vi "PID_Discipline_WithoutSystem_X72_Single.vi"(0 "SR620_No.1_Port":refnum<visa-resource-name>="GPIB0::20::INSTR", 1 "Channel (1: A)":i32(ring)=1 items=["Ext Input", "A", "B"], 2 "SR620_No.1 (1: REF)":i32(ring) items=["A", "B", "REF", "A / B"], 3 "Meas. Mode (0: Time)":i32(ring) items=["Time", "Width", "Rise / Fall Time", "Frequency", "Period", "Phase", "Count"], 4 "Arming Mode (0: +/-time)":i32(ring)=1 items=["+/-time", "+time", "1 period", "0.01s gate", "0.1s gate", "1.0s gate", "ext trig +/- time", "ext trig +time", "ext gate/+ time/hldf", "ext triggered 1 period", "ext triggered .01s gate", "ext triggered 0.1s gate", "ext triggered 1.0s gate"], 5 "Gate Time (Auto)":dbl(ring) items=["Auto"=0.0, "1E-6"=1e-06, "2E-6"=2e-06, "5E-6"=5e-06, "1E-5"=1e-05, "2E-5"=2e-05, "5E-5"=5e-05, "1E-4"=0.0001, "2E-4"=0.0002, "5E-4"=0.0005, "1E-3"=0.001, "2E-3"=0.002, "5E-3"=0.005, ".01"=0.01, ".02"=0.02, ".05"=0.05, ".1"=0.1, ".2"=0.2, ".5"=0.5, "1"=1.0, "2"=2.0, "5"=5.0, "10"=10.0, "20"=20.0, "50"=50.0, "100"=100.0, "200"=200.0, "500"=500.0], 6 "Sample Size (1)":u32(ring)=1 items=["1"=1, "2"=2, "5"=5, "10"=10, "20"=20, "50"=50, "100"=100, "200"=200, "500"=500, "1000"=1000, "2000"=2000, "5000"=5000, "10000"=10000, "20000"=20000, "50000"=50000, "100000"=100000, "200000"=200000, "500000"=500000, "1000000"=1000000], 7 "SR620_No.1_error in (no error)1":errorcluster, 8 "Input Termination_ (0: 50 Ohms)":i32(ring) items=["50 Ohms", "1 Mohm", "UHF Prescalers"], 9 "Timeout (25000 ms)":u32=1000 step=1000, 10 "Coupling (F: DC)":bool, 11 "Ref Out (1: TTL)":i32(ring)=1 items=["ECL", "TTL"], 12 "Auto Trigger Level (True)":bool, 14 "Trigger Level (0.00 V)":dbl=1.0, 16 "Trigger Slope (T: Positive)":bool=TRUE) -> (20 "SR620_No.1":refnum<visa-resource-name>="GPIB0::20::INSTR", 27 "SR620_No1 error out":errorcluster)   [LabVIEW 2014]
doc: "Provides an example of how to use the SR620 subVIs programmatically."
uses:
  <vilib>/addons/control/pid/pid.llb/PID (DBL).vi
  <vilib>/Utility/file.llb/Write To Spreadsheet File (DBL).vi
  <vilib>/Instr/_visa.llb/VISA Configure Serial Port (Instr).vi
  <vilib>/addons/control/pid/NI_PID_pid.lvlib
panel:
  out "本地测量钟差":dbl[](graph)=[7593300.0, 241.375901, 241.375903, 241.375876, 241.375868, 241.375803, 241.375857, 241.375887, 241.375852, 241.37583800000002, 241.37586299999998]
  in  "开始绘图":bool
  in  "delimiter (\\n)":string="\n" caption="数据分隔符(\\n)"
  in  "文件路径: single":path=path "C:/Users/Administrator/Desktop/PID_Discipline_WithoutSystem_X72_Single/single_read_data.txt"
  out "是否清零":dbl
  out "钟差改变量":dbl format="%#_10g"
  in  "驯服阈值(ns)":dbl=100.0
  out "驯服":bool
  out "当前粗调调整量（100ns）":i64
  in  "FPGA串口地址":refnum<visa-resource-name>="COM6"
  out "串口读取数值":i64
  out "读取缓冲区 （16进制）":string
  out "写入字符串2":string
  out "写入字符串1":string="0"
  out "最终粗调调整量（100ns）":i64
  in  "output range":cluster{"output high":dbl, "output low":dbl}={"output high"=400.0, "output low"=-400.0} caption="输出范围" {"output low" format="%.2f"; "output high" format="%.2f"}
  in  "PID gains":T1={"proportional gain (Kc)"=0.5, "integral time (Ti, min)"=0.0, "derivative time (Td, min)"=0.0} caption="PID增益" {"derivative time (Td, min)" format="%.3f"; "integral time (Ti, min)" format="%.3f"; "proportional gain (Kc)" format="%.3f"}
  out "反馈值":dbl format="%#.6f"
  in  "setpoint":dbl caption="设定值" format="%.3f"
  out "dt out (s)":dbl=1.0000000474974513 caption="dt输出(s)" format="%.3f"
  out "output":dbl caption="PID输出" format="%#.6f"
  in  "baud rate (9600) 2":u32=57600 caption="波特率(9600)"
  in  "VISA resource name 2":refnum<visa-resource-name>="COM3" caption="VISA资源名称"
  out "错误输出 2":errorcluster caption="错误输出"
  in  "baud rate (9600) 1":u32=57600 caption="波特率(9600)"
  in  "VISA resource name 1":refnum<visa-resource-name>="COM3" caption="VISA资源名称"
  out "错误输出 1":errorcluster caption="错误输出"
  out "串口工作":bool
  out "命令":string
  out "SR620_Delta_T":dbl format="%.12f"
  in  "等待时间（ms)":u32=1000
  out "总计数值":i32
  # "串口"
  # "数据处理"
  # "钟差调整量（ns）"
  # "数据显示及波形显示区域"
  # "公共调节区域"
  # "分别设置区域"
  # "Delta_T"
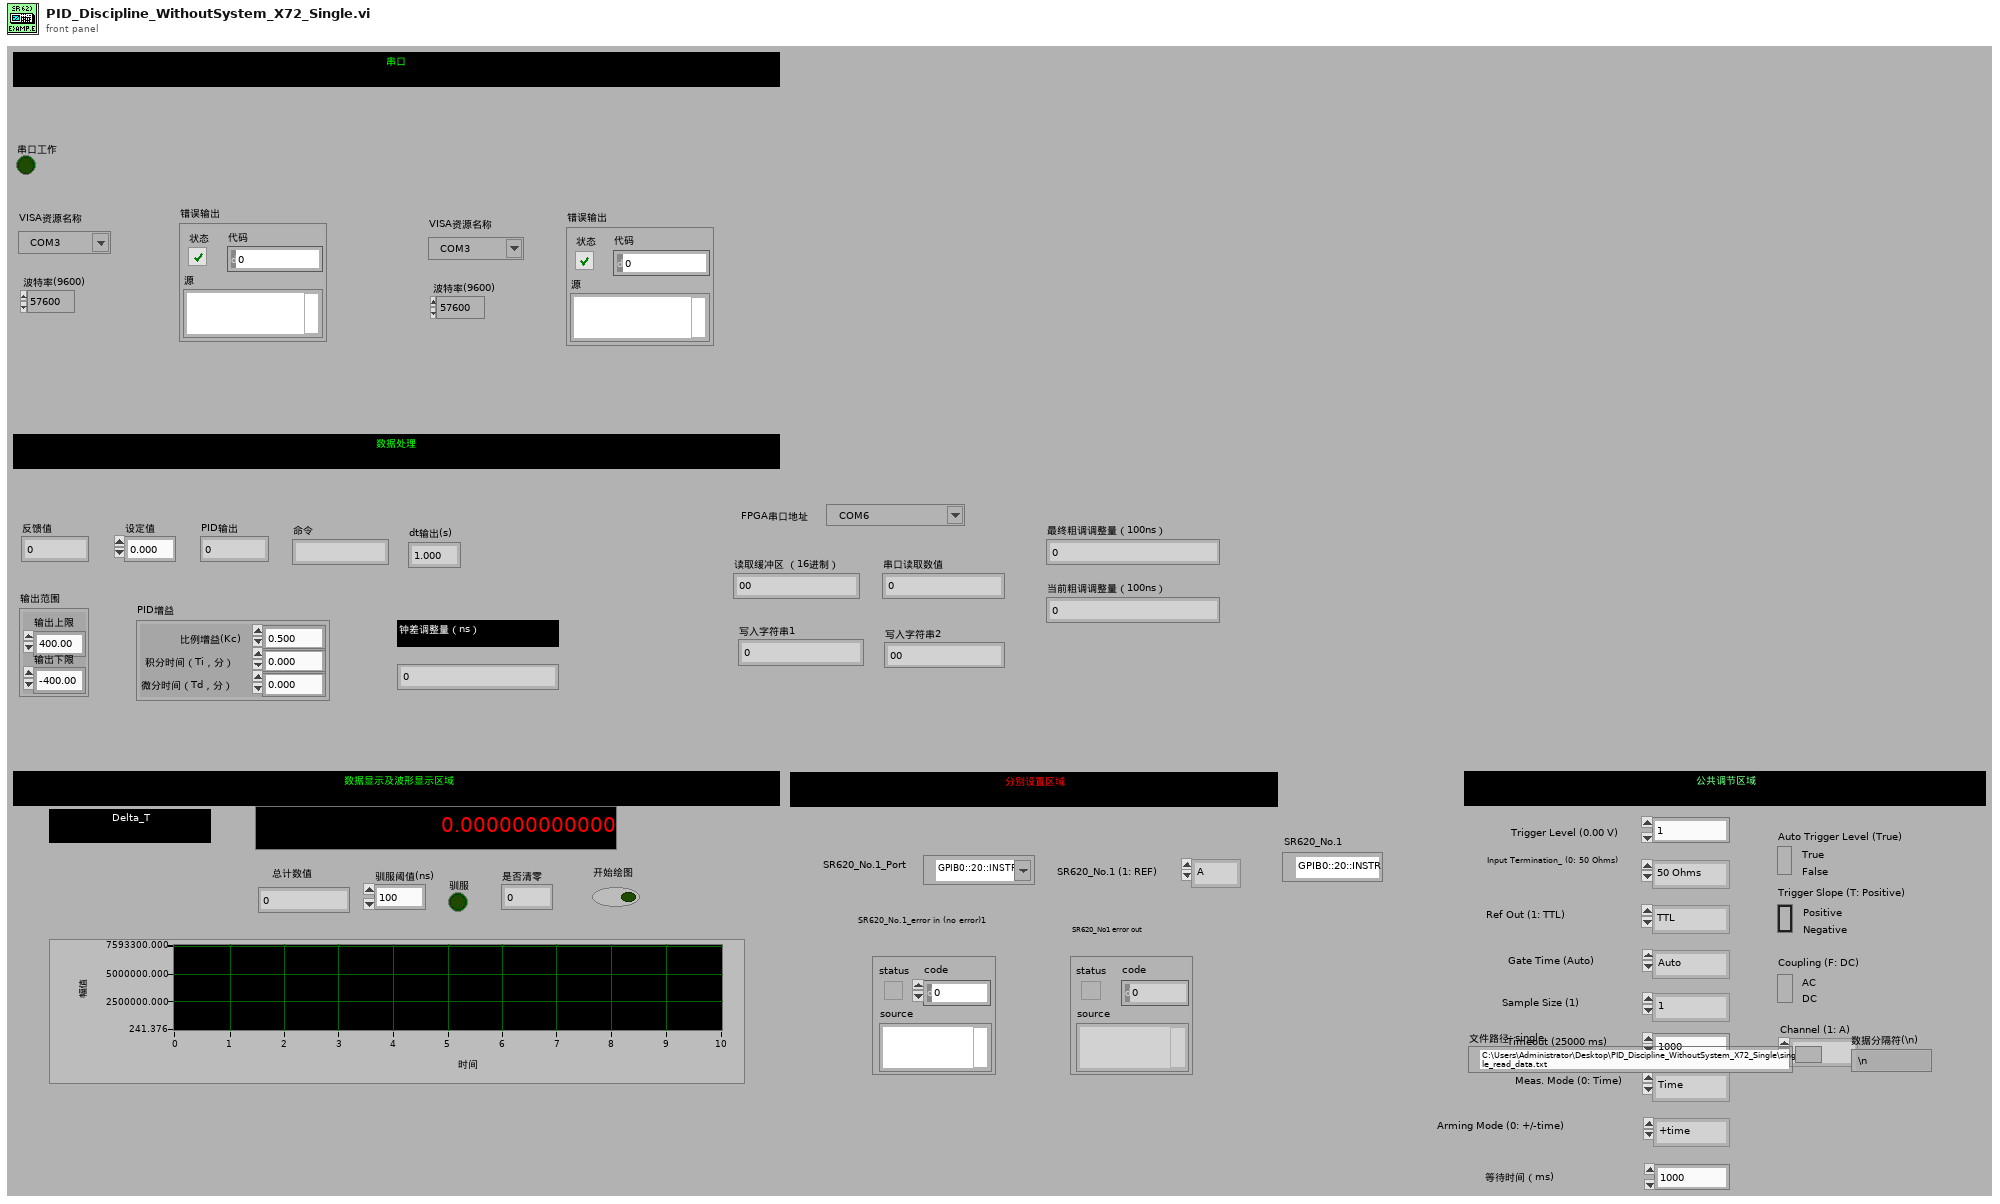
[diagram p1: front panel]
types:
  T1 = cluster{"proportional gain (Kc)":dbl, "integral time (Ti, min)":dbl, "derivative time (Td, min)":dbl}
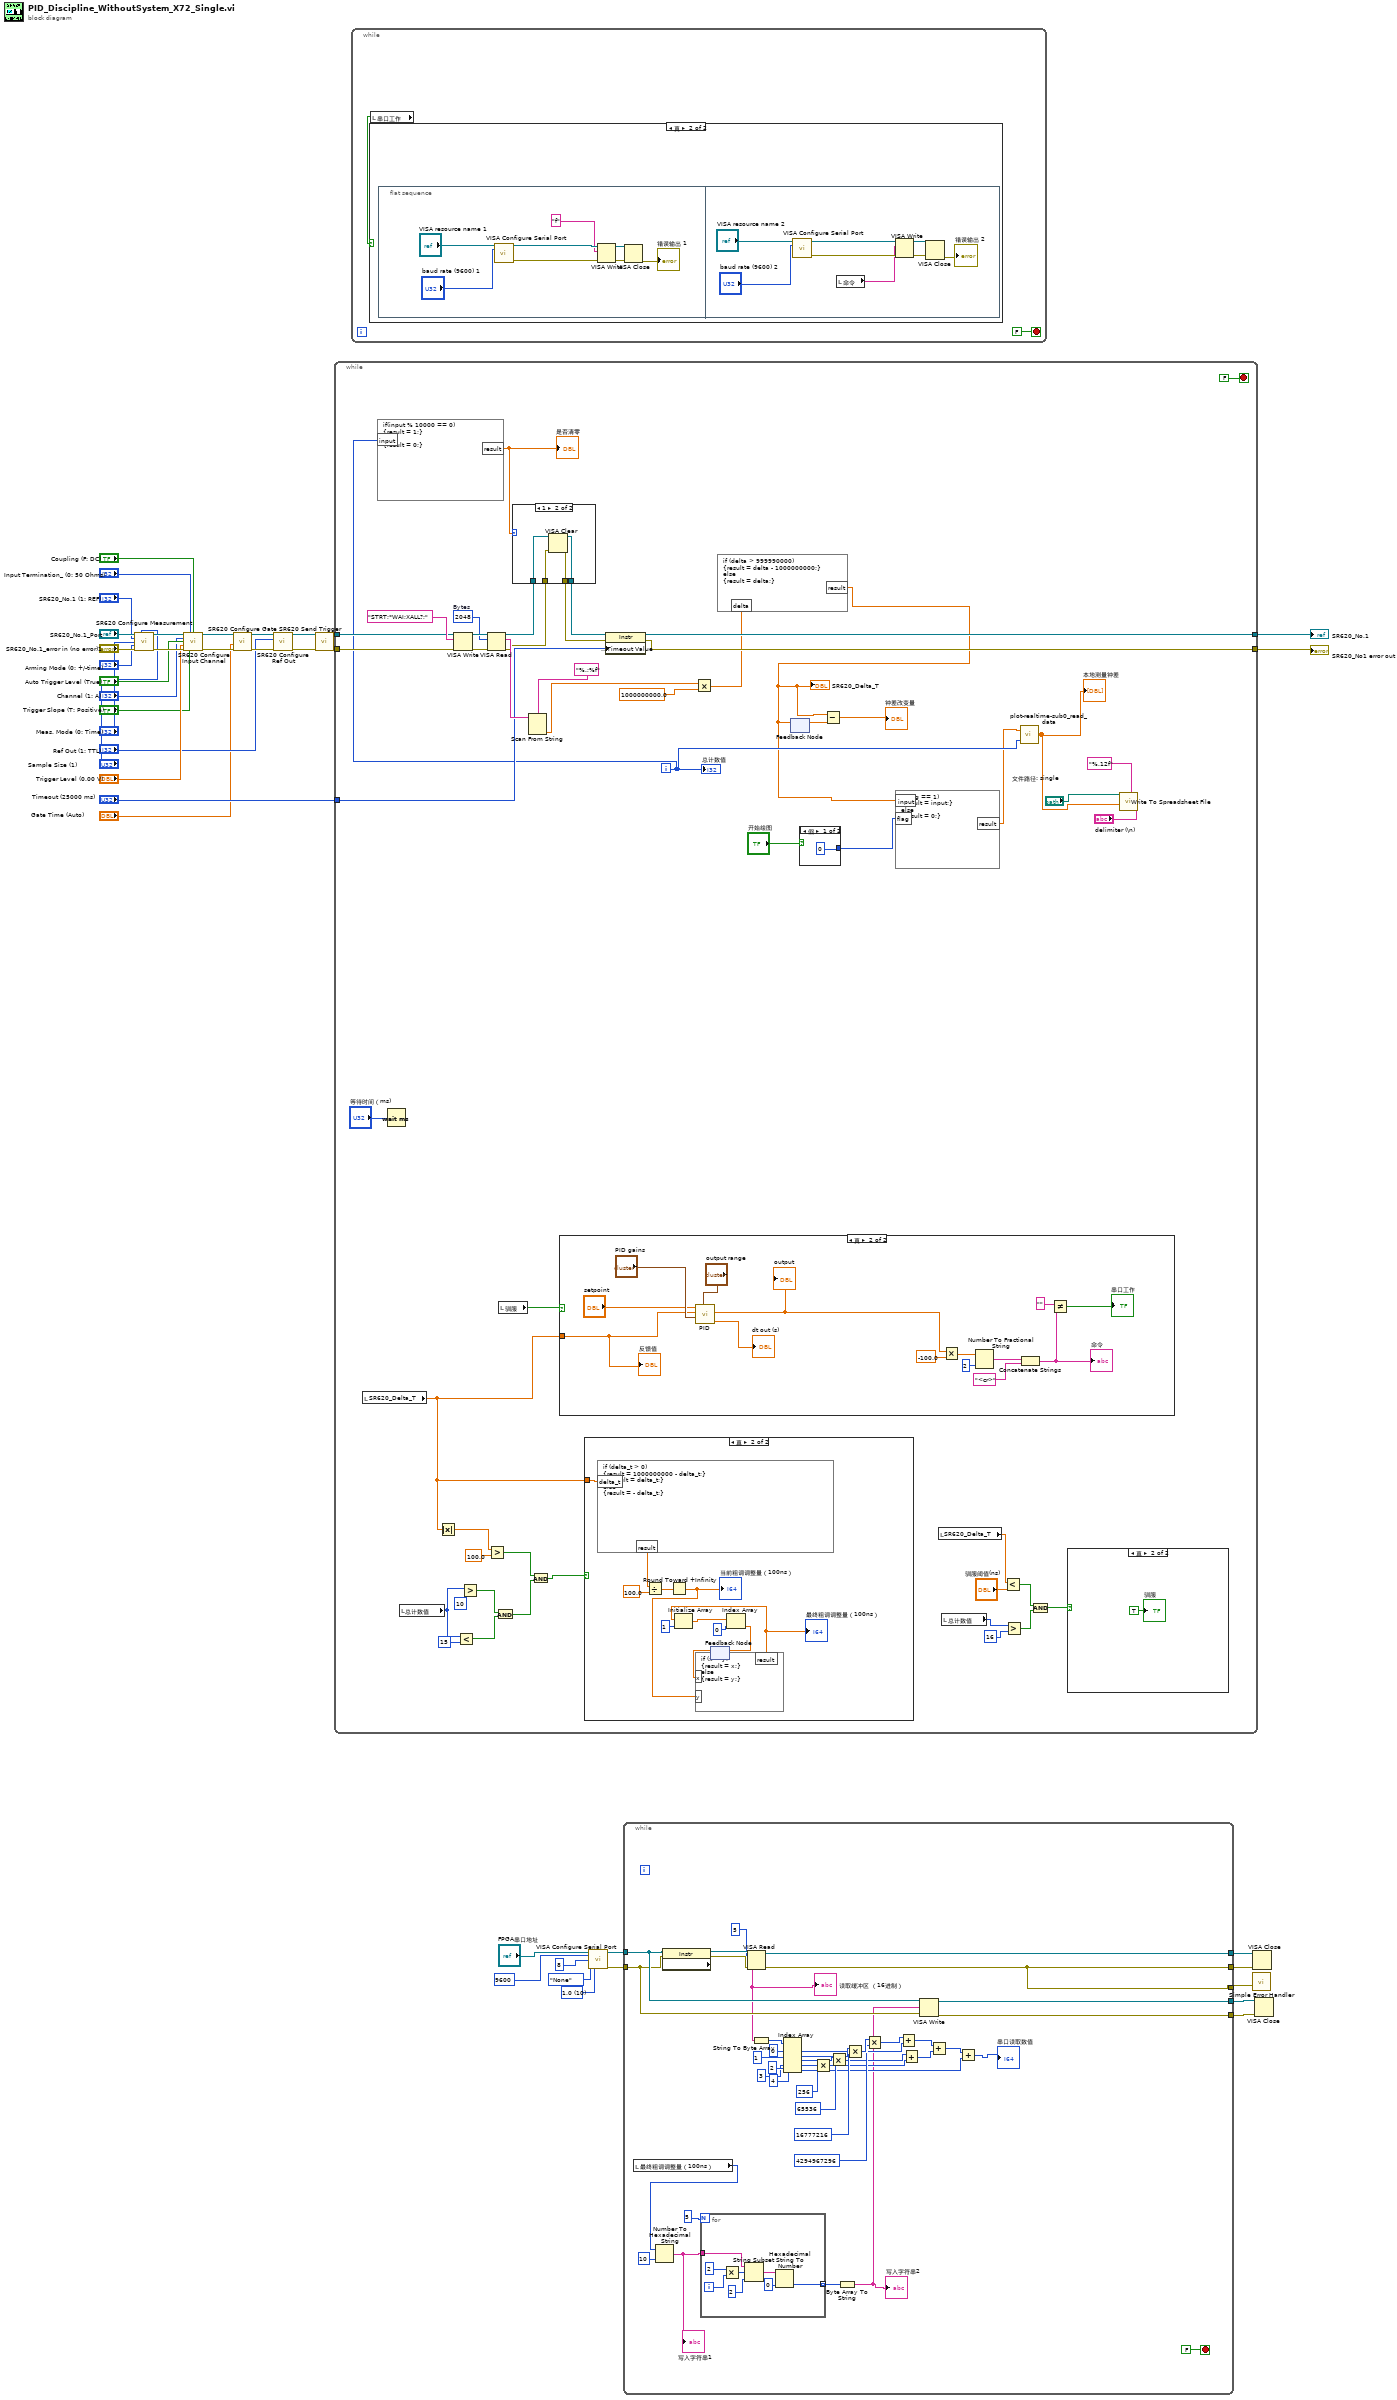
[diagram p0: block diagram]
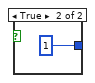
[diagram p3: hidden frame]
diagram:
  w20 = u16 10 items=["1.0"=10, "1.5"=15, "2.0"=20] ("stop bits (10: 1 bit)")
  n1 = call "SR620 Configure Measurement.vi"("VISA session"="SR620_No.1_Port", "Sample Size (1)"="Sample Size (1)", "Source (2: REF)"="SR620_No.1 (1: REF)", "Measurement Mode (0: Time)"="Meas. Mode (0: Time)", "Arming Mode (0: +/-time)"="Arming Mode (0: +/-time)", "error in (no error)"="SR620_No.1_error in (no error)1") -> ("dup VISA session"=w30:refnum<visa-resource-name>, "error out"=w28:errorcluster)  [unwired: 8 in]
  n2 = call "SR620 Configure Input Channel.vi"("VISA session"=w30, "Input Termination (0: 50 Ohms)"="Input Termination_ (0: 50 Ohms)", "Coupling (F: DC)"="Coupling (F: DC)", "Channel (1: A)"="Channel (1: A)", "Auto Trigger Level (True)"="Auto Trigger Level (True)", "Trigger Level (0.00 V)"="Trigger Level (0.00 V)", "error in (no error)"=w28, "Trigger Slope (T: Positive)"="Trigger Slope (T: Positive)") -> ("dup VISA session"=w29:refnum<visa-resource-name>, "error out"=w27:errorcluster)  [unwired: 6 in]
  n3 = call "SR620 Configure Gate.vi"("error in (no error)"=w27, "Gate Time (Auto)"="Gate Time (Auto)", "VISA session"=w29) -> ("error out"=w32:errorcluster, "dup VISA session"=w31:refnum<visa-resource-name>)  [unwired: 5 in]
  n4 = call "SR620 Configure Ref Out.vi"("error in (no error)"=w32, "Amplitude: Ref Output (1: TTL)"="Ref Out (1: TTL)", "VISA session"=w31) -> ("error out"=w33:errorcluster, "dup VISA session"=w34:refnum<visa-resource-name>)  [unwired: 3 in]
  n5 = call "SR620 Send Trigger.vi"("VISA session"=w34, "error in (no error)"=w33) -> ("dup VISA session"=w38:refnum<visa-resource-name>, "error out"=w37:errorcluster)  [unwired: 12 in]
  n6 = while "While循环" {
    tunnel: w38 -> [w84]
    tunnel: w37 -> [w83]
    tunnel: "Timeout (25000 ms)" -> [w60]
    tunnel: [w82] -> w25
    tunnel: [w81] -> w24
    i -> [w48]
    stop <- FALSE stop-if-true
    w88 = u32 2048  # Bytes
    n7 = local read "SR620_Delta_T"() -> (w55:dbl)
    n8 = formula code="if(input % 10000 == 0)\n{result = 1;}\nelse\n{result = 0;}"("input"=w48) -> ("result"=w49:dbl)
    "是否清零" <- w49
    n9 = Wait (ms)(milliseconds to wait="等待时间（ms)") -> ()  [unwired: 1 out]
    n10 = local read "总计数值"() -> (w75:i32)
    n11 = Absolute Value(x=w55) -> (abs(x)=w61:dbl)
    n12 = VISA Write(VISA resource name=w84, write buffer="STRT;*WAI;XALL?;" ("write buffer (\"\")"), error in (no error)=w83) -> (VISA resource name out=w89:refnum<visa-resource-name>, error out=w90:errorcluster)  [unwired: 1 out]
    n13 = Less?(x=w75, y=15) -> (x < y?=w72:bool)
    n14 = Greater?(x=w75, y=10) -> (0:w73:bool)
    n15 = VISA Read(VISA resource name=w89, byte count=w88, error in (no error)=w90) -> (VISA resource name out=w54:refnum<visa-resource-name>, read buffer=w85:string, error out=w52:errorcluster)  [unwired: 1 out]
    n16 = Greater?(x=w61, y=100.0) -> (0:w71:bool)
    n17 = And(x=w73, y=w72) -> (x .and. y?=w70:bool)
    n18 = local read "驯服"() -> (w63:bool)
    n19 = case shown="1" w49 {
      tunnel: w54 -> [w94 w98]
      tunnel: [w94 w97] -> w53
      tunnel: w52 -> [w93 w96]
      tunnel: [w93 w95] -> w51
      frame 0, Default {
      }
      frame 1 {
        n20 = VISA Clear(VISA resource name=w98, error in (no error)=w96) -> (VISA resource name out=w97:refnum<visa-resource-name>, error out=w95:errorcluster)
      }
    }
    n21 = Scan From String(format string="%.;%f", input string=w85) -> (output 1=w79:dbl)  [unwired: 3 in, 3 out]
    n22 = And(x=w71, y=w70) -> (x .and. y?=w69:bool)
    n23 = case shown="真" w63 {
      tunnel: w55 -> [_ w120]
      frame False {
      }
      frame True {
        n24 = call-poly <vilib>:"PID.vi"("output range"="output range", "PID gains"="PID gains", "process variable"=w120, "setpoint"="setpoint") -> ("dt out (s)"=→"dt out (s)":dbl, "output"=w112:dbl)  [unwired: 6 in]
        "output" <- w112
        n25 = Multiply(x=w112, y=-100.0) -> (x*y=w111:dbl)
        n26 = Number To Fractional String(number=w111, precision (6)=i16 2 ("精度(6)")) -> (F-format string=w118:string)  [unwired: 2 in]
        n27 = Concatenate Strings(w118, "<cr>" ("字符串")) -> (w114:string)
        "命令" <- w114
        n28 = Not Equal?(x="", y=w114) -> (x != y?=→"串口工作":bool)
        "反馈值" <- w120
      }
    }
    n29 = case shown="真" w69 {
      tunnel: w55 -> [_ w100]
      frame False {
      }
      frame True {
        n30 = formula code="if (delta_t > 0)\n{result = 1000000000 - delta_t;}\n//{result = delta_t;}\nelse\n{result = - delta_t;}"("delta_t"=w100) -> ("result"=w109:dbl)
        n31 = Divide(x=w109, y=100.0) -> (x/y=w108:dbl)
        n32 = Round Toward +Infinity(x=w108) -> (ceil(x): smallest int >= x=w102:dbl)
        "当前粗调调整量（100ns）" <- w102
        n33 = feedback #1() -> (w103:dbl)  [unwired: 1 in]
        n34 = formula code="if (x > y)\n{result = x;}\nelse\n{result = y;}"("x"=w103, "y"=w102) -> ("result"=w101:dbl)
        "最终粗调调整量（100ns）" <- w101
        n35 = Initialize Array(w101, 1 ("维数大小")) -> (w105:dbl[])
        n36 = Index Array(array=w105, index=0 ("索引")) -> (element=w104:dbl)
        n37 = feedback-in #1(w104) -> ()
      }
    }
    n38 = property class="Instr"(reference=w53, error in=w51, "General Settings:Timeout Value"=w60) -> (reference out=w82:refnum<visa-resource-name>, error out=w81:errorcluster)
    n39 = Multiply(x=w79, y=1000000000.0) -> (x*y=w56:dbl)
    n40 = formula code="if (delta > 999990000)\n{result = delta - 1000000000;}\nelse\n{result = delta;}"("delta"=w56) -> ("result"=w44:dbl)
    "SR620_Delta_T" <- w44
    n41 = feedback #2() -> (w59:dbl)  [unwired: 1 in]
    n42 = feedback-in #2(w44) -> ()
    n43 = case shown="假" "开始绘图" {
      tunnel: [0 1] -> w42
      frame False {
      }
      frame True {
      }
    }
    n44 = Subtract(x=w44, y=w59) -> (x-y=→"钟差改变量":dbl)
    n45 = formula code="if(flag == 1)\n{result = input;}\nelse\n{result = 0;}"("flag"=w42, "input"=w44) -> ("result"=w41:dbl)
    n46 = local read "SR620_Delta_T"() -> (w57:dbl)
    n47 = local read "总计数值"() -> (w68:i32)
    n48 = Less?(x=w57, y="驯服阈值(ns)") -> (x < y?=w66:bool)
    n49 = Greater?(x=w68, y=16) -> (0:w65:bool)
    n50 = call "plot-realtime-sub0_read_data.vi"("索引"=w48, "x"=w41) -> ("数组"=w40:dbl[])
    "本地测量钟差" <- w40
    n51 = And(x=w66, y=w65) -> (x .and. y?=w64:bool)
    n52 = case shown="真" w64 {
      frame False {
      }
      frame True {
        "驯服" <- TRUE
      }
    }
    n53 = call-poly <vilib>:"Write To Spreadsheet File.vi"("delimiter (\\t)"="delimiter (\\n)", "format (%.3f)"="%.12f", "1D data"=w40, "file path (dialog if empty)"="文件路径: single") -> ()  [unwired: 4 in, 1 out]
    "总计数值" <- w48
  }
  "SR620_No.1" <- w25
  "SR620_No1 error out" <- w24
  n54 = while {
    stop <- FALSE stop-if-true
    n55 = local read "串口工作"() -> (w125:bool)
    n56 = case shown="真" w125 {
      frame False {
      }
      frame True {
        n57 = flat-sequence {
          frame #0 {
            n58 = call-poly "VISA Configure Serial Port"("VISA resource name"="VISA resource name 1", "baud rate (9600)"="baud rate (9600) 1") -> ("VISA resource name out"=w134:refnum<visa-resource-name>, "error out"=w131:errorcluster)  [unwired: 12 in]
            n59 = VISA Write(VISA resource name=w134, write buffer="f" ("写入缓冲区"), error in (no error)=w131) -> (VISA resource name out=w129:refnum<visa-resource-name>, error out=w128:errorcluster)  [unwired: 1 out]
            n60 = VISA Close(VISA resource name=w129, error in (no error)=w128) -> (error out=→"错误输出 1":errorcluster)
          }
          frame #1 {
            n61 = call-poly "VISA Configure Serial Port"("VISA resource name"="VISA resource name 2", "baud rate (9600)"="baud rate (9600) 2") -> ("VISA resource name out"=w139:refnum<visa-resource-name>, "error out"=w141:errorcluster)  [unwired: 12 in]
            n62 = local read "命令"() -> (w138:string)
            n63 = VISA Write(VISA resource name=w139, write buffer=w138, error in (no error)=w141) -> (VISA resource name out=w137:refnum<visa-resource-name>, error out=w136:errorcluster)  [unwired: 1 out]
            n64 = VISA Close(VISA resource name=w137, error in (no error)=w136) -> (error out=→"错误输出 2":errorcluster)
          }
        }
      }
    }
  }
  n65 = call-poly "VISA Configure Serial Port"("VISA resource name"="FPGA串口地址", "baud rate (9600)"=u32 9600, "data bits (8)"=u16 8, "parity (0:none)"=enum16{"None", "Odd", "Even", "Mark", "Space"}."None", "stop bits (10: 1 bit)"=w20) -> ("VISA resource name out"=w18:refnum<visa-resource-name>, "error out"=w17:errorcluster)  [unwired: 9 in]
  n66 = while {
    tunnel: w18 -> [w180]
    tunnel: w17 -> [w179]
    tunnel: [w177] -> w16
    tunnel: [w176] -> w15
    tunnel: [w176] -> w14
    tunnel: [w175] -> w13
    tunnel: [w174] -> w12
    stop <- FALSE stop-if-true
    n67 = local read "最终粗调调整量（100ns）"() -> (w144:i64)
    n68 = Number To Hexadecimal String(1:i16 10 ("宽度(-)"), 2:w144) -> (0:w146:string)
    "写入字符串1" <- w146
    n69 = property class="Instr" props=["Serial Settings:Number of Bytes at Serial Port"](reference=w180, error in=w179) -> (reference out=w182:refnum<visa-resource-name>, error out=w181:errorcluster)  [unwired: 1 out]
    n70 = for {
      N: 5 -> [_]
      tunnel: w146 -> [w186]
      tunnel: [w183] -> w148 mode=indexing
      i -> [w190]
      n71 = Multiply(x=2, y=w190) -> (x*y=w188:i32)
      n72 = String Subset(string=w186, offset (0)=w188, length (rest)=2) -> (substring=w185:string)
      n73 = Hexadecimal String To Number(string=w185, default (0uL)=u8 0 ("默认(0 U32)")) -> (number=w183:u8)  [unwired: 1 in, 1 out]
    }
    n74 = VISA Read(VISA resource name=w182, byte count=5, error in (no error)=w181) -> (VISA resource name out=w177:refnum<visa-resource-name>, read buffer=w150:string, error out=w176:errorcluster)  [unwired: 1 out]
    "读取缓冲区 （16进制）" <- w150
    n75 = String To Byte Array(string=w150) -> (unsigned byte array=w173:u8[])
    n76 = Index Array ("索引数组")(array=w173, index #1=0 ("索引"), index #2=1 ("索引"), index #3=2 ("索引"), index #4=3 ("索引"), index #5=4 ("索引")) -> (element #1=w161:u8, element #2=w162:u8, element #3=w164:u8, element #4=w165:u8, element #5=w152:u8)
    n77 = Multiply ("乘")(x=w165, y=i64 256) -> (x*y=w156:i64)
    n78 = Multiply ("乘")(x=w164, y=i64 65536) -> (x*y=w157:i64)
    n79 = Byte Array To String(unsigned byte array=w148) -> (string=w145:string)
    "写入字符串2" <- w145
    n80 = Multiply ("乘")(x=w162, y=i64 16777216) -> (x*y=w158:i64)
    n81 = Multiply ("乘")(x=w161, y=i64 4294967296) -> (x*y=w159:i64)
    n82 = Add ("加")(x=w159, y=w158) -> (x+y=w155:i64)
    n83 = Add ("加")(x=w157, y=w156) -> (x+y=w154:i64)
    n84 = VISA Write(VISA resource name=w180, write buffer=w145, error in (no error)=w179) -> (VISA resource name out=w175:refnum<visa-resource-name>, error out=w174:errorcluster)  [unwired: 1 out]
    n85 = Add ("加")(x=w155, y=w154) -> (x+y=w153:i64)
    n86 = Add ("加")(x=w153, y=w152) -> (x+y=→"串口读取数值":i64)
  }
  n87 = call <vilib>:"Simple Error Handler.vi"("error in (no error)"=w14) -> ()  [unwired: 4 in, 5 out]
  n88 = VISA Close(VISA resource name=w16, error in (no error)=w15) -> ()  [unwired: 1 out]
  n89 = VISA Close(VISA resource name=w13, error in (no error)=w12) -> ()  [unwired: 1 out]
